vi "defaultConfiguration.vi"(8 "error in (no error)":errorcluster, 11 "Camera in":refnum<class "Camera.lvclass">) -> (0 "error out":errorcluster, 3 "Camera out":refnum<class "Camera.lvclass">)   [LabVIEW 2019, in "Camera.lvclass"]
doc: "Sets the camera to it’s default configuration. This function is also called during initialization inside\ninit.vi"
uses:
  Camera.lvclass
  Camera.lvclass/Camera.ctl
  pco.sdk/RecordingControl/RecordingControl.lvlib
  pco.sdk/GeneralCameraControl/GeneralCameraControl.lvlib
  pco.sdk/ImageInformation/ImageInformation.lvlib
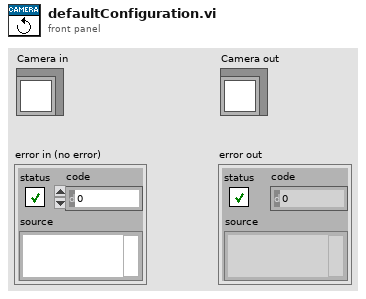
[diagram p1: front panel]
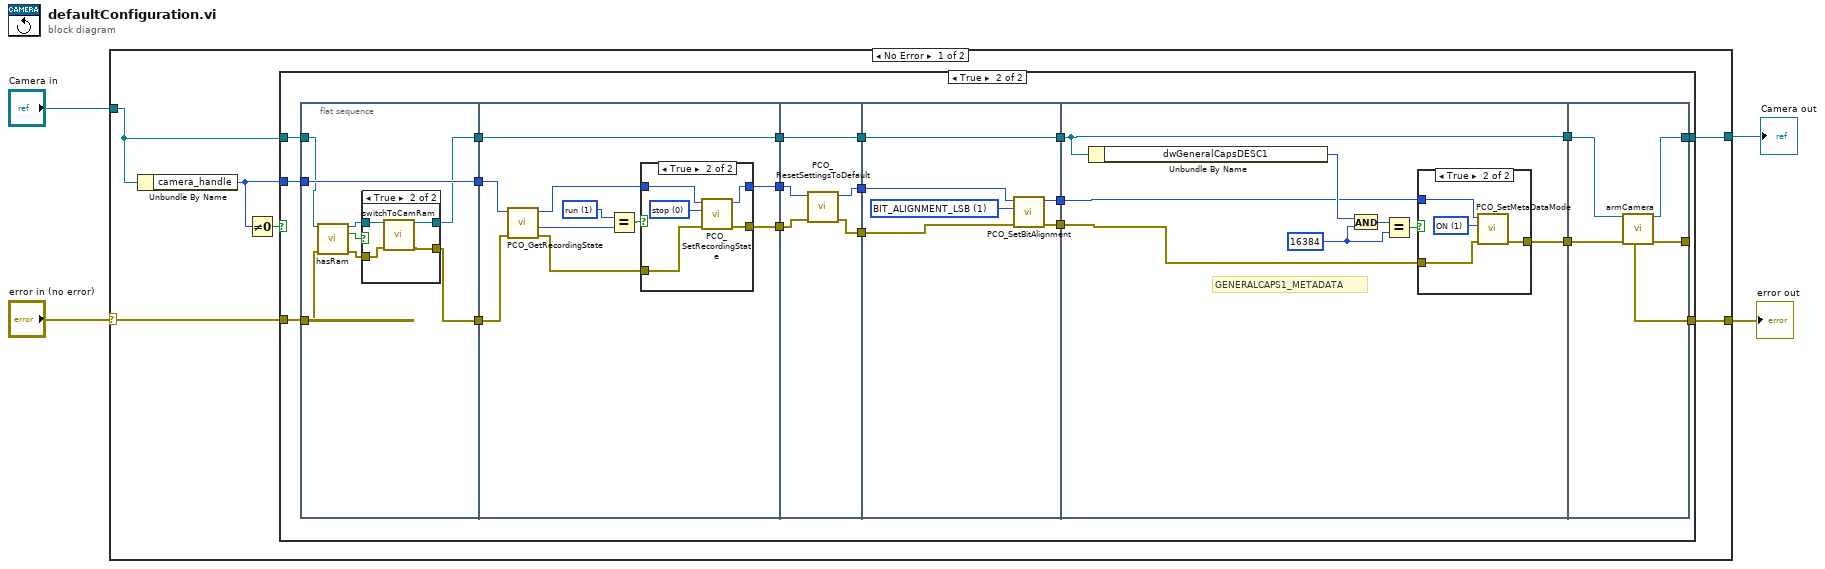
[diagram p0: block diagram]
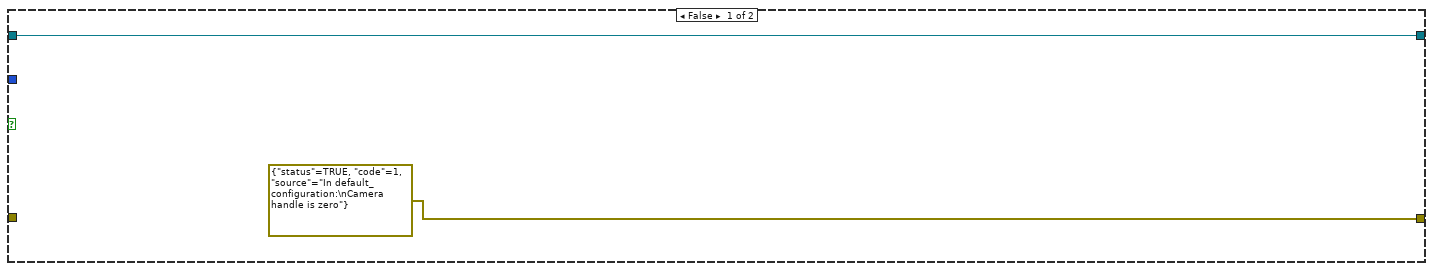
[diagram p2: hidden frame]
diagram:
  n1 = case shown="No Error" "error in (no error)" {
    selector: "error in (no error)" -> [w8 w92]
    tunnel: [w7 w92] -> w3
    tunnel: [w5 w91] -> w1
    tunnel: "Camera in" -> [w6 w91]
    frame No Error {
      n2 = Unbundle By Name(w6) -> ("camera_handle"=w9:u64)
      n3 = Not Equal To 0?(x=w9) -> (x != 0?=w10:bool)
      n4 = case shown="True" w10 {
        tunnel: [errorcluster {"status"=TRUE, "code"=1, "source"="In default_configuration:\nCamera handle is zero"} ("error constant") w17] -> w7
        tunnel: w9 -> [_ w30]
        tunnel: w8 -> [_ w31]
        tunnel: w6 -> [w11 w22]
        tunnel: [w11 w13] -> w5
        frame False {
        }
        frame True {
          n5 = flat-sequence {
            tunnel: w22 -> [w37]
            tunnel: w30 -> [w39]
            tunnel: w31 -> [w35]
            tunnel: [w33] -> w16
            tunnel: [w39] -> w15
            tunnel: [w32] -> w14
            tunnel: [w49] -> w29
            tunnel: [w47] -> w28
            tunnel: [w46] -> w23
            tunnel: w16 -> [w55]
            tunnel: w15 -> [w54]
            tunnel: w14 -> [w46]
            tunnel: w29 -> [w67]
            tunnel: w28 -> [w66]
            tunnel: [w65] -> w27
            tunnel: [w64] -> w26
            tunnel: w23 -> [w63]
            tunnel: [w63] -> w20
            tunnel: w27 -> [w73]
            tunnel: w26 -> [w72]
            tunnel: [w71] -> w25
            tunnel: [w70] -> w24
            tunnel: [w69] -> w21
            tunnel: w20 -> [w69]
            tunnel: w25 -> [w76]
            tunnel: w24 -> [w77]
            tunnel: w21 -> [w74]
            tunnel: [w75] -> w19
            tunnel: [w74] -> w18
            tunnel: [w90] -> w17
            tunnel: w19 -> [w89]
            tunnel: w18 -> [w88]
            tunnel: [w87] -> w13
            frame #0 {
              n6 = call-dynamic "hasRam.vi"("Camera in"=w37, "error in (no error)"=w35) -> ("Camera out"=w36:refnum<class "Camera.lvclass">, "hasRam"=w38:bool, "error out"=w34:errorcluster)  [unwired: 11 in]
              n7 = case shown="True" w38 {
                tunnel: w36 -> [w41 w45]
                tunnel: w34 -> [w40 w44]
                tunnel: [w40 w43] -> w33
                tunnel: [w41 w42] -> w32
                frame False {
                }
                frame True {
                  n8 = call-dynamic "switchToCamRam.vi"("Camera in"=w45, "error in (no error)"=w44) -> ("Camera out"=w42:refnum<class "Camera.lvclass">, "error out"=w43:errorcluster)  [unwired: 12 in]
                }
              }
            }
            frame #1 {
              w52 = u16 1 items=["stop", "run"] ("wRecState")
              n9 = call "PCO_GetRecordingState.vi"("error in (no error)"=w55, "ph"=w54) -> ("error out"=w50:errorcluster, "wRecState"=w53:u16, "ph out"=w48:u64)  [unwired: 6 in, 1 out]
              n10 = Equal?(x=w52, y=w53) -> (x = y?=w51:bool)
              n11 = case shown="True" w51 {
                tunnel: w50 -> [w57 w61]
                tunnel: [w57 w60] -> w49
                tunnel: w48 -> [w56 w59]
                tunnel: [w56 w58] -> w47
                frame False {
                }
                frame True {
                  w62 = u16 0 items=["stop", "run"] ("wRecState")
                  n12 = call "PCO_SetRecordingState.vi"("error in (no error)"=w61, "wRecState"=w62, "ph"=w59) -> ("error out"=w60:errorcluster, "ph out"=w58:u64)  [unwired: 6 in, 1 out]
                }
              }
            }
            frame #2 {
              n13 = call "PCO_ResetSettingsToDefault.vi"("error in (no error)"=w67, "ph"=w66) -> ("error out"=w65:errorcluster, "ph out"=w64:u64)  [unwired: 7 in, 1 out]
            }
            frame #3 {
              w68 = u16 1 items=["BIT_ALIGNMENT_MSB", "BIT_ALIGNMENT_LSB"] ("wBitAlignment")
              n14 = call "PCO_SetBitAlignment.vi"("error in (no error)"=w73, "wBitAlignment"=w68, "ph"=w72) -> ("error out"=w70:errorcluster, "ph out"=w71:u64)  [unwired: 6 in, 1 out]
            }
            frame #4 {
              w80 = u32 16384 ("y")
              # "GENERALCAPS1_METADATA"
              n15 = Unbundle By Name(w74) -> ("dwGeneralCapsDESC1"=w78:u32)
              n16 = And(x=w78, y=w80) -> (x .and. y?=w81:u32)
              n17 = Equal?(x=w81, y=w80) -> (x = y?=w79:bool)
              n18 = case shown="True" w79 {
                tunnel: w77 -> [w82 w84]
                tunnel: w76 -> [_ w85]
                tunnel: [w82 w83] -> w75
                frame False {
                }
                frame True {
                  w86 = u16 1 items=["OFF", "ON"] ("wMetaDataMode")
                  n19 = call "PCO_SetMetaDataMode.vi"("error in (no error)"=w84, "wMetaDataMode"=w86, "ph"=w85) -> ("error out"=w83:errorcluster)  [unwired: 4 in, 4 out]
                }
              }
            }
            frame #5 {
              n20 = call-dynamic "armCamera.vi"("Camera in"=w88, "error in (no error)"=w89) -> ("Camera out"=w87:refnum<class "Camera.lvclass">, "error out"=w90:errorcluster)  [unwired: 12 in]
            }
          }
        }
      }
    }
    frame Error {
    }
  }
  "error out" <- w3
  "Camera out" <- w1
